vi "PAN_PostCommand.vi"(4 "Modules":string[](array[string])=["GUNSC", "GFITS", "LOGIC", "BUFMGR"], 5 "cmdQ":refnum<queue>, 6 "queue out":refnum<queue>, 7 "command":string, 8 "error in (no error)":errorcluster, 9 "timeout":u32, 10 "orig exptime":dbl format="%.2f", 11 "DHE_DBSRef":T3) -> (0 "error out":errorcluster, 2 "exp time":dbl format="%.2f")   [LabVIEW 2016]
uses:
  Modules/DBSHAND/private/vis/DatabaseHand_RefNum.ctl
  PAN_actionsSTruct.ctl
  PAN_cmdStruct.ctl
  Modules/DBSHAND/private/vis/DatabaseHand_Element_Get(bool).vi
panel:
  in  "cmd struct":T1
  in  "action struct":T2
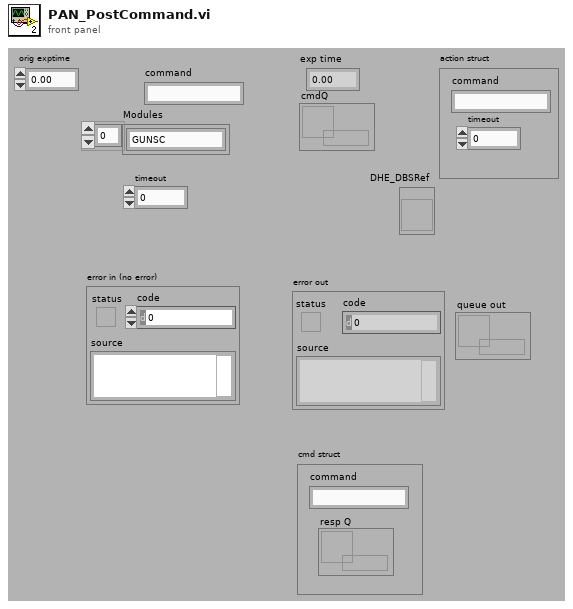
[diagram p1: front panel]
types:
  T1 = typedef "PAN_cmdStruct.ctl" = cluster{"command":string, "resp Q":refnum<queue>}
  T2 = typedef "PAN_actionsSTruct.ctl" = cluster{"command":string, "timeout":u32}
  T3 = typedef "DatabaseHand_RefNum.ctl" = refnum<vi>
  T4 = enum16{"add", "delete", "clean", "shutdown", "hold", "continue", "modify"}
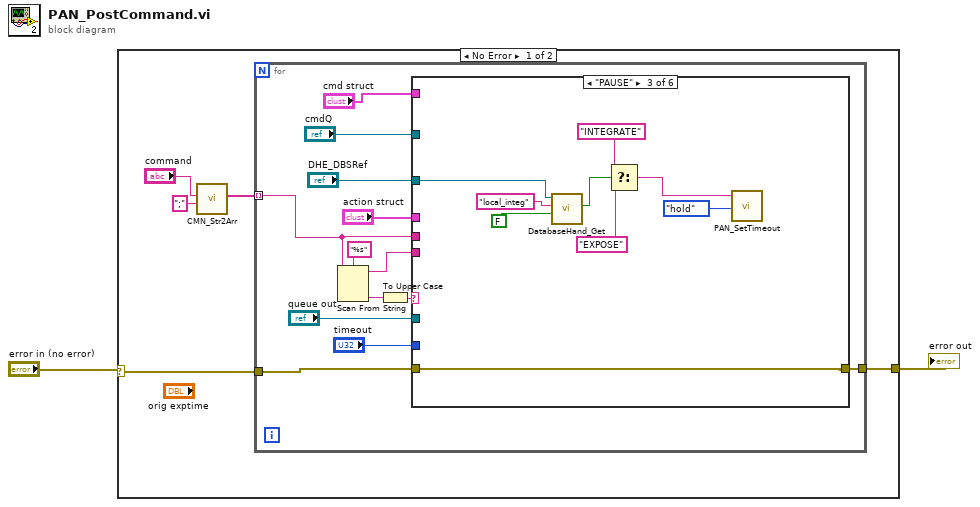
[diagram p0: block diagram]
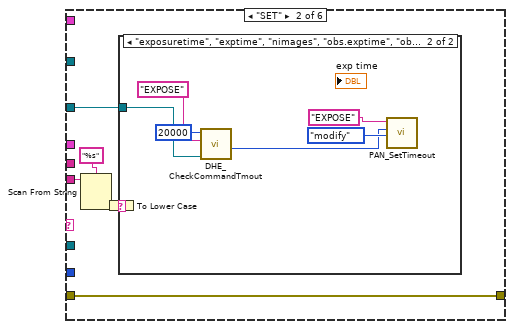
[diagram p3: hidden frame]
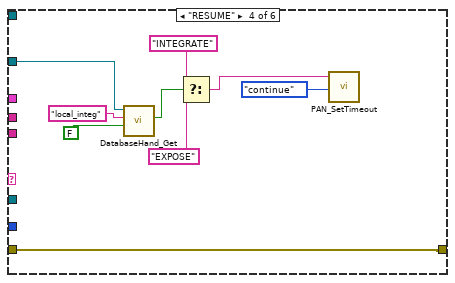
[diagram p5: hidden frame]
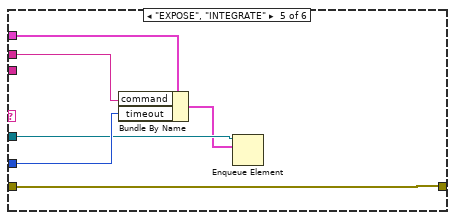
[diagram p6: hidden frame]
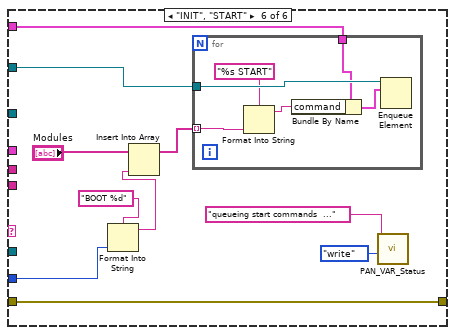
[diagram p7: hidden frame]
diagram:
  n1 = case shown="No Error" "error in (no error)" {
    selector: "error in (no error)" -> [w6 w74]
    tunnel: [w7 w74] -> w2
    frame No Error {
      n2 = call "CMN_Str2Arr.vi"("separator"=";", "string in"="command") -> ("Array out"=w3:string[])  [unwired: 2 in, 7 out]
      n3 = for {
        tunnel: [w18] -> w7
        tunnel: w6 -> [w16]
        tunnel: w3 -> [w9] mode=indexing
        n4 = Scan From String(format string="%s", input string=w9) -> (remaining string=w8:string, output 1=w20:string)  [unwired: 2 in, 3 out]
        n5 = To Upper Case(1:w20) -> (0:w15:string)
        n6 = case shown="\"PAUSE\"" w15 {
          tunnel: w16 -> [w21 w27 w41 w50 w57 w67]
          tunnel: [w21 w27 w41 w50 w57 w67] -> w18
          tunnel: "DHE_DBSRef" -> [_ w26 w39 w43 _ _]
          tunnel: "timeout" -> [_ _ _ _ w56 w62]
          tunnel: "queue out" -> [_ _ _ _ w55 _]
          tunnel: "action struct" -> [_ _ _ _ w53 _]
          tunnel: w9 -> [_ _ _ _ w52 _]
          tunnel: "cmdQ" -> [_ _ _ _ _ w66]
          tunnel: "cmd struct" -> [_ _ _ _ _ w63]
          tunnel: w8 -> [_ w25 _ _ _ _]
          frame Default {
          }
          frame "SET" {
            n7 = Scan From String(format string="%s", input string=w25) -> (output 1=w23:string)  [unwired: 2 in, 4 out]
            n8 = To Lower Case(string=w23) -> (all lower case string=w22:string)
            n9 = case shown="\"exposuretime\", \"exptime\", \"nimages\", \"obs.exptime\", \"obs.nimages\", \"obs.numreads\"" w22 {
              tunnel: w26 -> [_ w31]
              frame Default {
              }
              frame "exposuretime", "exptime", "nimages", "obs.exptime", "obs.nimages", "obs.numreads" {
                n10 = call "DHE_CheckCommandTmout.vi"("DBSRef"=w31, "Command"="EXPOSE", "TimeOut in"=20000) -> ("TimeOut out"=w28:i32)  [unwired: 2 in, 5 out]
                n11 = call "PAN_SetTimeout.vi"("action"=T4."modify", "timeout"=w28, "Command"="EXPOSE") -> ()  [unwired: 1 in, 8 out]
              }
            }
          }
          frame "PAUSE" {
            n12 = call-poly "DatabaseHand_Get.vi"("default value"=FALSE, "name"="local_integ", "Database RefNum in"=w39) -> ("value"=w37:bool)  [unwired: 2 in, 6 out]
            n13 = Select(t="INTEGRATE", s=w37, f="EXPOSE" ("Command")) -> (s? t:f=w35:string)
            n14 = call "PAN_SetTimeout.vi"("action"=T4."hold", "Command"=w35) -> ()  [unwired: 2 in, 8 out]
          }
          frame "RESUME" {
            n15 = call-poly "DatabaseHand_Get.vi"("default value"=FALSE, "name"="local_integ", "Database RefNum in"=w43) -> ("value"=w47:bool)  [unwired: 2 in, 6 out]
            n16 = Select(t="INTEGRATE", s=w47, f="EXPOSE" ("Command")) -> (s? t:f=w44:string)
            n17 = call "PAN_SetTimeout.vi"("action"=T4."continue", "Command"=w44) -> ()  [unwired: 2 in, 8 out]
          }
          frame "EXPOSE", "INTEGRATE" {
            n18 = Bundle By Name(cluster=w53, "command"=w52, "timeout"=w56) -> (w54:T2)
            n19 = Enqueue Element(queue=w55, element=w54) -> ()  [unwired: 1 in, 4 out]
          }
          frame "INIT", "START" {
            n20 = Format Into String(format string="BOOT %d" ("new element/subarray"), w62) -> (resulting string=w60:string)  [unwired: 2 in, 1 out]
            n21 = Insert Into Array(array="Modules", new element=w60) -> (w64:string[])  [unwired: 1 in]
            n22 = for {
              tunnel: w66 -> [w73]
              tunnel: w64 -> [w70] mode=indexing
              tunnel: w63 -> [w68]
              n23 = Format Into String(format string="%s START", w70) -> (resulting string=w69:string)  [unwired: 2 in, 1 out]
              n24 = Bundle By Name(cluster=w68, "command"=w69) -> (w72:T1)
              n25 = Enqueue Element(queue=w73, element=w72) -> ()  [unwired: 1 in, 4 out]
            }
            n26 = call "PAN_VAR_Status.vi"("action"=enum16{"read", "write", "set_ref"}."write", "status in"="queueing start commands  ...") -> ()  [unwired: 2 in, 8 out]
          }
        }
      }
    }
    frame Error {
    }
  }
  "error out" <- w2
